vi "Drive Modifications.vi"(1 "Drive Global Data In":T1) -> (0 "Drive Global Data Out":T1)   [LabVIEW 2013]
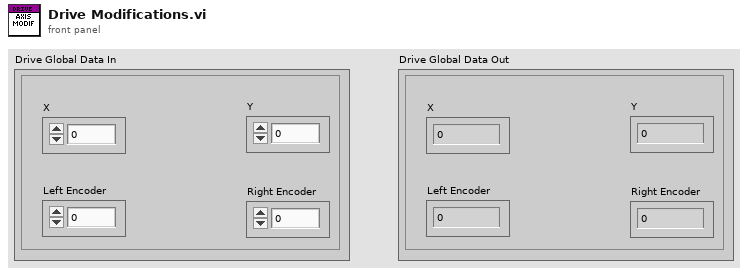
[diagram p1: front panel]
types:
  T1 = cluster{"Y":dbl, "X":dbl, "Left Encoder":dbl, "Right Encoder":dbl}
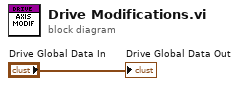
[diagram p0: block diagram]
diagram:
  "Drive Global Data Out" <- "Drive Global Data In"
